vi "Example-tagDisplayContainer.vi"() -> ()   [LabVIEW 2020]
uses:
  639bab4c-25e0-41ff-b8d6-0a38394ec7c6.vi
  <userlib>/_NEVSTOP/TagDB/_Support/DataAccess/data-Write.vi
  <userlib>/_NEVSTOP/TagDB/_Support/URL/TRIM-BOTH-SPACE.vi
  <userlib>/_NEVSTOP/TagDB/_Support/Error/_[error50000]Invalid DB REF.vi
  <userlib>/_NEVSTOP/TagDB/_Support/DataAccess/TagDB Ref to DVR.vi
  <userlib>/_NEVSTOP/TagDB/_Support/DataAccess/_NameCacher.vi
  <userlib>/_NEVSTOP/TagDB/_Support/DataAccess/_datatypeChecker.vi
  <vilib>/Utility/Data Type/Get Type Information.vi
  <userlib>/_NEVSTOP/TagDB/_Support/Error/_Build Error Cluster.vi
  <userlib>/_NEVSTOP/TagDB/Add-ons/RefManager/_Support/UISync/_Pull Controls Value to DPs(VI).vi
  <userlib>/_NEVSTOP/TagDB/TagDB.lvlib
  <userlib>/_NEVSTOP/Communicable State Machine(CSM)/Communicable State Machine.lvlib
  TagDashboard/CSM-TagDashboard.lvlib
  <userlib>/_NEVSTOP/TagDB/Add-ons/RefManager/TagDB RefManager.lvlib
  TagDisplayContainer/CSM-TagDBDisplayContainer.lvlib
  392d5714-9003-442d-ab5f-f13be5cc2abb.vi
panel:
  in  "被试泵#3":dbl
  in  "被试泵#2":dbl
  in  "被试泵#1":dbl
  in  "API: Switch >> SubVIEW2 -@ ViewContainer":bool
  in  "API: Switch >> SubVIEW1 -@ ViewContainer":bool
  in  "stop":bool
  in  "高温泵压力#3":dbl
  in  "高温泵压力#2":dbl
  in  "高温泵压力#1":dbl
  in  "被试泵流量#3":dbl
  in  "被试泵流量#2":dbl
  in  "被试泵流量#1":dbl
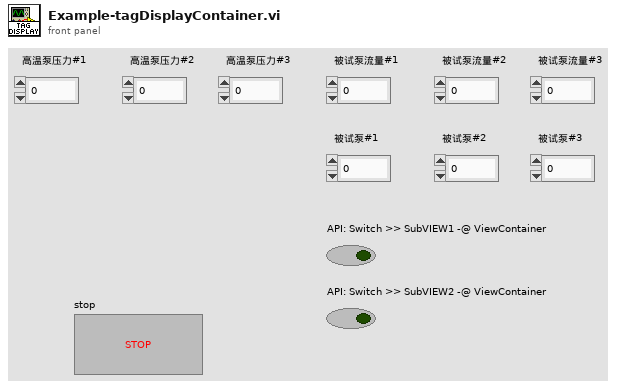
[diagram p1: front panel]
types:
  T1 = cluster{"高温泵压力#2":dbl, "高温泵压力#1":dbl, "高温泵压力#3":dbl, "被试泵流量#3":dbl, "被试泵流量#2":dbl, "被试泵流量#1":dbl, "被试泵#3":dbl, "被试泵#2":dbl, "被试泵#1":dbl}
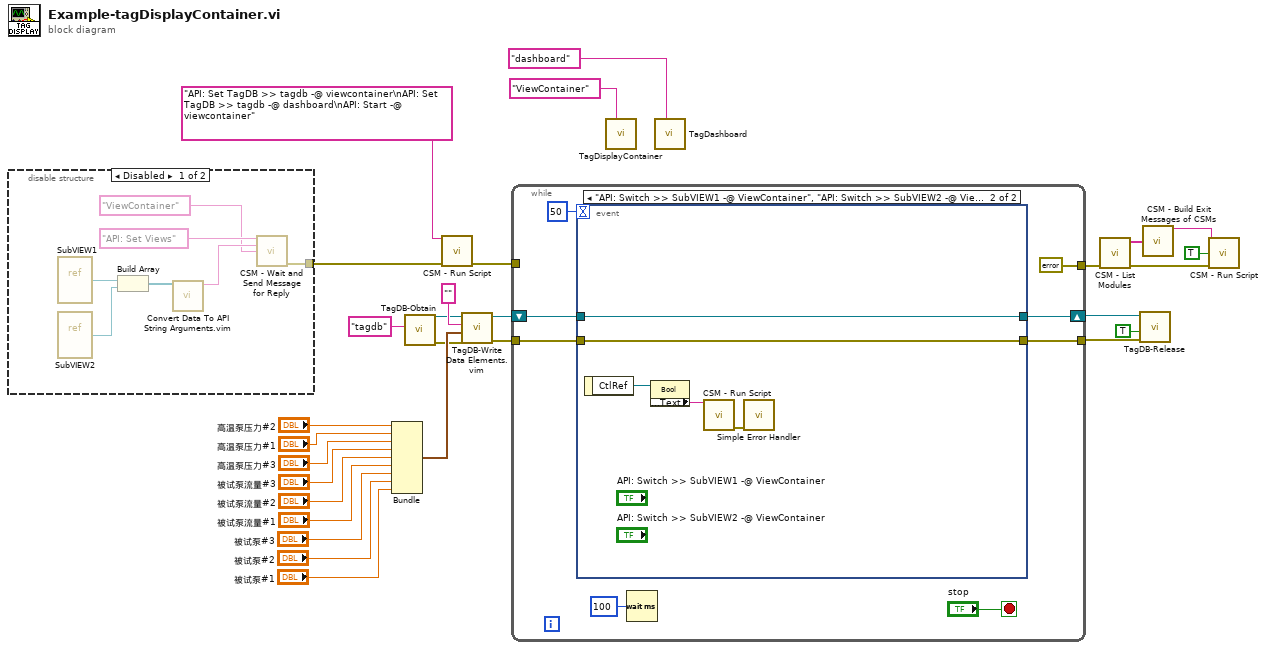
[diagram p0: block diagram]
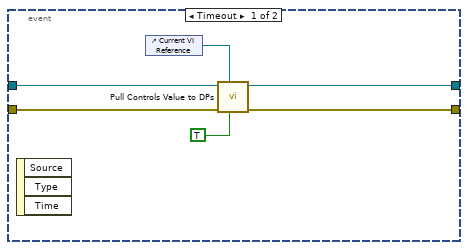
[diagram p3: hidden frame]
diagram:
  n1 = disable-structure shown="Disabled" {
    disable-tunnel: [w34 _] -> w29
    frame Disabled {
      n2 = vi-ref "SubVIEW1.vi"() -> (w32:refnum<vi>)
      n3 = vi-ref "SubVIEW2.vi"() -> (w30:refnum<vi>)
      n4 = Build Array(w32, w30) -> (w31:refnum<vi>[])
      n5 = call "Convert Data To API String Arguments.vim"("Data"=w31) -> ("API String"=w35:string)  [unwired: 7 in, 1 out]
      n6 = call <userlib>:"CSM - Wait and Send Message for Reply.vi"("State"="API: Set Views", "Arguments (\"\")"=w35, "Target Module"="ViewContainer" ("Name (\"\" to Use UUID)")) -> ("error out"=w34:errorcluster)  [unwired: 9 in, 3 out]
    }
    frame Enabled {
    }
  }
  n7 = Bundle("高温泵压力#2"="高温泵压力#2", "高温泵压力#1"="高温泵压力#1", "高温泵压力#3"="高温泵压力#3", "被试泵流量#3"="被试泵流量#3", "被试泵流量#2"="被试泵流量#2", "被试泵流量#1"="被试泵流量#1", "被试泵#3"="被试泵#3", "被试泵#2"="被试泵#2", "被试泵#1"="被试泵#1") -> (w13:T1)  [unwired: 1 in]
  n8 = call <userlib>:"TagDB-Obtain.vi"("name (unnamed)"="tagdb") -> ("error out"=w5:errorcluster, "TagDB"=w4:refnum<k1>)  [unwired: 4 in, 1 out]
  n9 = call <userlib>:"CSM - Run Script.vi"("CSM Scripts"="API: Set TagDB >> tagdb -@ viewcontainer\nAPI: Set TagDB >> tagdb -@ dashboard\nAPI: Start -@ viewcontainer", "error in (no error)"=w29) -> ("error out"=w27:errorcluster)  [unwired: 11 in, 2 out]
  n10 = call "TagDB-Write Data Elements.vim"("error in (no error)"=w5, "Value"=w13, "Root Tag(\"\")"="" ("root tag"), "TagDB"=w4) -> ("error out"=w2:errorcluster, "TagDB(dup)"=w3:refnum<k1>)  [unwired: 5 in, 1 out]
  n11 = while {
    tunnel: w27 -> [_]
    shift-right: [w42] -> w26
    shift-left: w3 -> [w43]
    tunnel: w2 -> [w41]
    tunnel: [w40] -> w25
    tunnel: [errorcluster {"status"=FALSE, "code"=0, "source"=""} ("Error In (No Error)")] -> w17
    stop <- "stop" stop-if-true
    n12 = event shown="[1] \"API: Switch >> SubVIEW1 -@ ViewContainer\", \"API: Switch >> SubVIEW2 -@ ViewContainer\": Value Change" {
      selector: _ -> [_ _]
      dyn-events: _ -> [_ _]
      timeout: 50 -> [_ _]
      tunnel: w43 -> [w49 w51]
      tunnel: [w48 w51] -> w42
      tunnel: w41 -> [w50 w52]
      tunnel: [w47 w52] -> w40
      event Timeout {
        n13 = event-data() -> ()  [unwired: 1 in, 3 out]
        n14 = control-ref of="Current VI Reference"() -> (w45:refnum<vi>)
        n15 = call-poly <userlib>:"Pull Controls Value to DPs.vi"("sync DPs?(T)"=TRUE, "VIRef(Caller VI)"=w45, "error in (no error)"=w50, "SILAPI In"=w49) -> ("error out"=w47:errorcluster, "SILAPI Out"=w48:refnum<k1>)  [unwired: 5 in, 1 out]
      }
      event "API: Switch >> SubVIEW1 -@ ViewContainer", "API: Switch >> SubVIEW2 -@ ViewContainer": Value Change {
        n16 = event-data() -> ("CtlRef"=w55:refnum<vi>)  [unwired: 1 in]
        n17 = property class="Bool"(reference=w55) -> ("Label.Text"=w54:string)  [unwired: 1 in, 2 out]
        n18 = call <userlib>:"CSM - Run Script.vi"("CSM Scripts"=w54) -> ("error out"=w53:errorcluster)  [unwired: 12 in, 2 out]
        n19 = call <vilib>:"Simple Error Handler.vi"("error in (no error)"=w53) -> ()  [unwired: 4 in, 5 out]
      }
    }
    n20 = Wait (ms)(milliseconds to wait=u32 100) -> ()  [unwired: 1 out]
  }
  n21 = call "TagDisplayContainer.vi"("Name(\"\" to use uuid)"="ViewContainer" ("Name (\"\" to Use UUID)")) -> ()  [unwired: 11 in]
  n22 = call "TagDashboard.vi"("Name(\"\" to use uuid)"="dashboard" ("Name(\"\" to use uuid)")) -> ()  [unwired: 11 in]
  n23 = call <userlib>:"CSM - List Modules.vi"("Error In"=w17) -> ("error out"=w21:errorcluster, "Module Names"=w19:string[])  [unwired: 9 in]
  n24 = call <userlib>:"TagDB-Release.vi"("error in (no error)"=w25, "force destroy? (F)"=TRUE, "TagDB"=w26) -> ()  [unwired: 8 in, 1 out]
  n25 = call <userlib>:"CSM - Build Exit Messages of CSMs.vi"("CSMs"=w19) -> ("States"=w20:string)  [unwired: 14 in]
  n26 = call <userlib>:"CSM - Run Script.vi"("CSM Scripts"=w20, "Continue If Error? (F)"=TRUE, "error in (no error)"=w21) -> ()  [unwired: 10 in, 3 out]
